vi "Sweep Step.vi"(8 "error in (no error)":errorcluster, 11 "Power Supply in":refnum<class "Power Supply.lvclass">) -> (0 "error out":errorcluster, 1 "Done?":bool, 2 "field":dbl[unit], 3 "Power Supply out":refnum<class "Power Supply.lvclass">, 4 "rate":dbl[unit])   [LabVIEW 2009, in "Power Supply.lvclass"]
doc: "As the field sweeps, monitor that the current sweep rate is still appropriate and adjust as necessary."
uses:
  Power Supply.lvclass
  Ramping Mode.ctl
  Power Supply.lvclass/Power Supply.ctl
panel:
  in  "Ramping Mode":T1
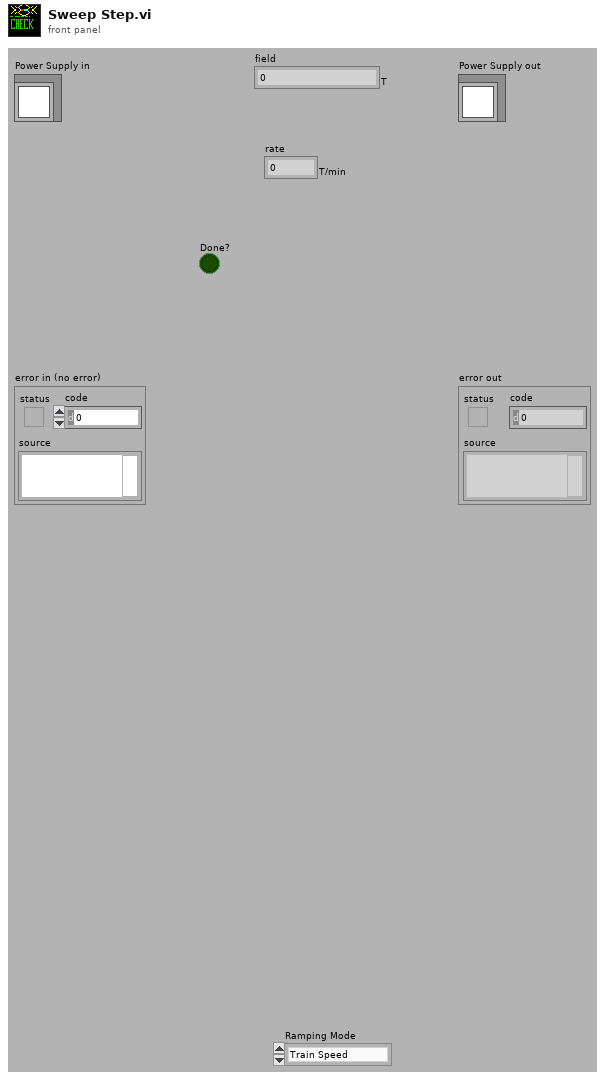
[diagram p1: front panel]
types:
  T1 = typedef "Power Supply.lvclass/Ramping Mode.ctl" = enum16{"Train Speed", "Maximum Speed", "Manual"}
  T2 = typedef "PSIO.ctl" = cluster{"Address":T3, "Version":enum16{"PS", "IPS"}}
  T3 = typedef "OxfordAddress.ctl" = cluster{"Com Port":i32, "ISOBUS Address":i32, "GPIB Address":i16, "Communication":enum16{"RS232", "ISOBUS", "GPIB", "Gateway"}}
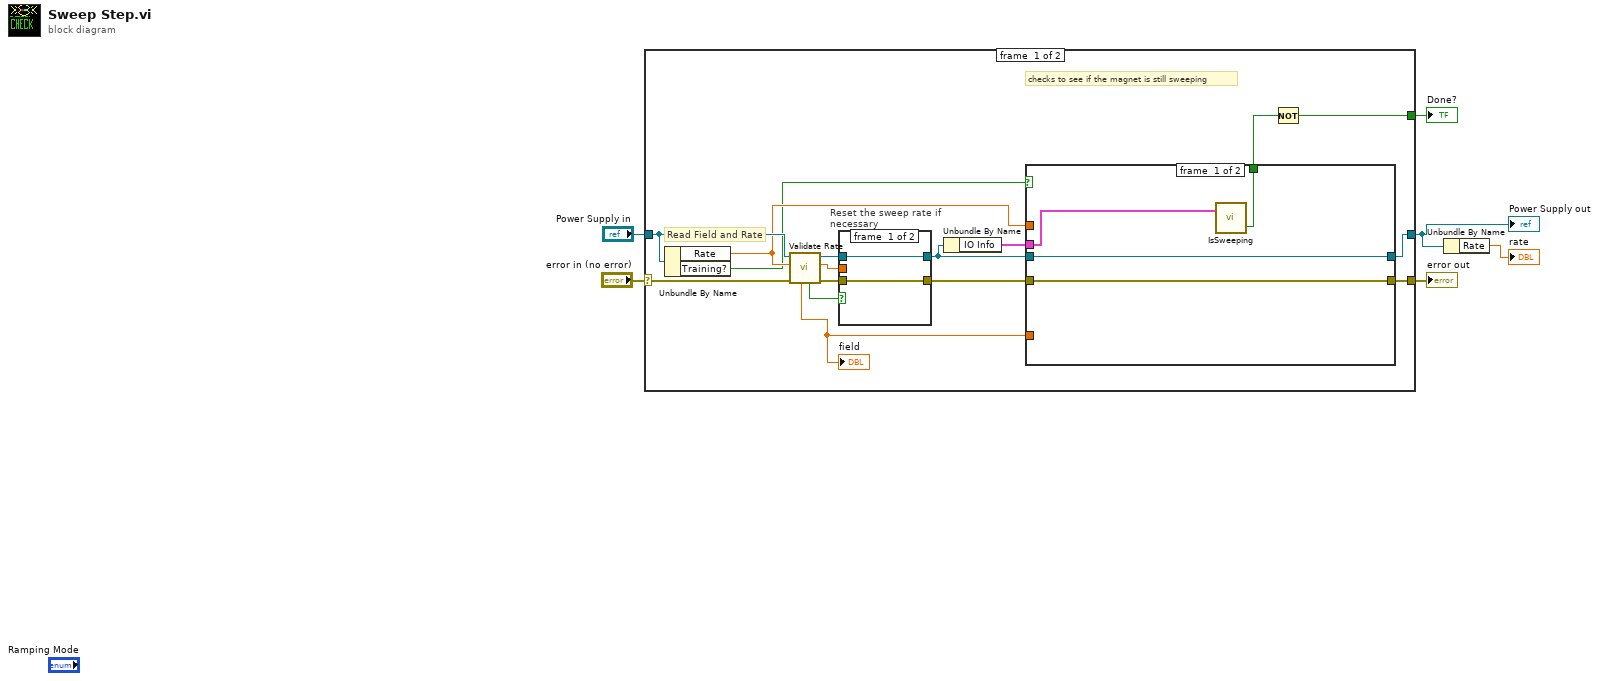
[diagram p0: block diagram]
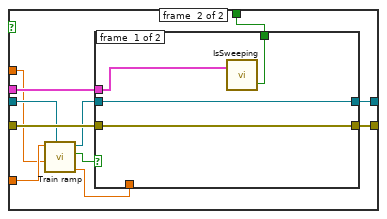
[diagram p2: hidden frame]
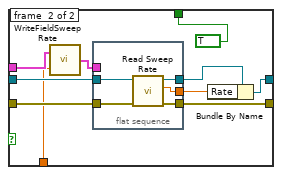
[diagram p3: hidden frame]
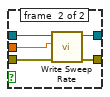
[diagram p4: hidden frame]
diagram:
  n1 = case shown="No Error" "error in (no error)" {
    selector: "error in (no error)" -> [w19 w64]
    tunnel: [w18 _] -> w6
    tunnel: [w16 w64] -> w5
    tunnel: [w12 w65] -> w2
    tunnel: "Power Supply in" -> [w20 w65]
    frame #0 {
      # "checks to see if the magnet is still sweeping"
      # "Read Field and Rate"
      n2 = Unbundle By Name(w20) -> ("Rate"=w9:dbl[unit], "Training?"=w8:bool)
      n3 = call "Validate Rate.vi"("error IO"=w19, "rate"=w9, "Power Supply in"=w20) -> ("error out"=w22:errorcluster, "Coerced rate"=w14:dbl[unit], "Power Supply out"=w21:refnum<class "Power Supply.lvclass">, "Coerced?"=w11:bool, "Field"=w10:dbl[unit])  [unwired: 3 in, 1 out]
      "field" <- w10
      n4 = case "Reset the sweep rate if necessary" shown="True" w11 {
        tunnel: w14 -> [_ w61]
        tunnel: w22 -> [w57 w63]
        tunnel: [w57 w62] -> w17
        tunnel: w21 -> [w58 w60]
        tunnel: [w58 w59] -> w13
        frame #0 {
        }
        frame #1 {
          n5 = call-dynamic "Write Sweep Rate.vi"("error in (no error)"=w63, "rate"=w61, "Power Supply in"=w60) -> ("error out"=w62:errorcluster, "Power Supply out"=w59:refnum<class "Power Supply.lvclass">)  [unwired: 7 in]
        }
      }
      n6 = Unbundle By Name(w13) -> ("IO Info"=w15:T2)
      n7 = case shown="True" w8 {
        tunnel: w17 -> [w25 w37]
        tunnel: [w25 w36] -> w16
        tunnel: w15 -> [w24 w34]
        tunnel: w13 -> [w26 w30]
        tunnel: [w26 w35] -> w12
        tunnel: w10 -> [_ w28]
        tunnel: w9 -> [_ w27]
        tunnel: [w23 w33] -> w7
        frame #0 {
          n8 = call "IsSweeping.vi"("IO Info"=w24) -> ("Sweeping"=w23:bool)  [unwired: 2 out]
        }
        frame #1 {
          n9 = call "Train ramp.vi"("pwr supply in"=w30, "input"=w27, "field"=w28) -> ("output"=w31:dbl[unit], "change?"=w32:bool, "pwr supply out"=w29:refnum<class "Power Supply.lvclass">)  [unwired: 6 in]
          n10 = case shown="True" w32 {
            tunnel: w37 -> [w40 w49]
            tunnel: [w40 w48] -> w36
            tunnel: w29 -> [w41 w47]
            tunnel: [w41 w46] -> w35
            tunnel: w34 -> [w39 w45]
            tunnel: [w38 TRUE] -> w33
            tunnel: w31 -> [_ w42]
            frame #0 {
              n11 = call "IsSweeping.vi"("IO Info"=w39) -> ("Sweeping"=w38:bool)  [unwired: 2 out]
            }
            frame #1 {
              n12 = call "WriteFieldSweepRate.vi"("Sweep rate"=w42, "IO Info"=w45) -> ("IO Info"=w50:T2)
              n13 = flat-sequence {
                tunnel: [w56] -> w44
                tunnel: w47 -> [w55]
                tunnel: [w54] -> w51
                tunnel: w50 -> [_]
                tunnel: w49 -> [w53]
                tunnel: [w52] -> w48
                frame #0 {
                  n14 = call-dynamic "Read Sweep Rate.vi"("error in (no error)"=w53, "Power Supply in"=w55) -> ("error out"=w52:errorcluster, "Field sweep rate"=w56:dbl[unit], "Power Supply out"=w54:refnum<class "Power Supply.lvclass">)  [unwired: 7 in]
                }
              }
              n15 = Bundle By Name(cluster=w51, "Rate"=w44) -> (w46:refnum<class "Power Supply.lvclass">)
            }
          }
        }
      }
      n16 = Not(x=w7) -> (.not. x?=w18:bool)
    }
    frame #1 {
    }
  }
  "Done?" <- w6
  "error out" <- w5
  "Power Supply out" <- w2
  n17 = Unbundle By Name(w2) -> ("Rate"=→"rate":dbl[unit])
